vi "找搜索线上的分界点.vi"(6 "圆心":cluster{"X":sgl, "Y":sgl}, 9 "ROI 找边":T1 {"Contours"."Type" items=["No Selection", "Point", "Line", "Rectangle", "Oval", "Polygon", "Freehand Region", "Annulus", "Unused2", "Unused3", "Broken Line", "Freehand Line", "Rotated Rectangle"]}, 10 "Options":T3={"Edge Polarity"=2, "Kernel Size"=7, "Width"=7, "Minimum Edge Strength"=20.0, "Interpolation Type"=enum."Bilinear Fixed", "Data Processing Method"=enum."Average"} {"Edge Polarity" items=["All Edges", "Rising Edges", "Falling Edges"]; "Minimum Edge Strength" format="%.2f"; "Width" step=2; "Kernel Size" step=2}, 11 "引用句柄输入":T2) -> (0 "两点之间距离":sgl, 2 "Location (Pixel)":cluster{"X":sgl, "Y":sgl}, 3 "引用句柄输出":T2)   [LabVIEW 2014]
uses:
  <vilib>/vision/Measure.llb/Edge Options.ctl
  <vilib>/vision/Measure.llb/Edge Polarity.ctl
  <vilib>/vision/Image Controls.llb/IMAQ Image.ctl
  <vilib>/vision/NI_Vision_Development_Module.lvlib
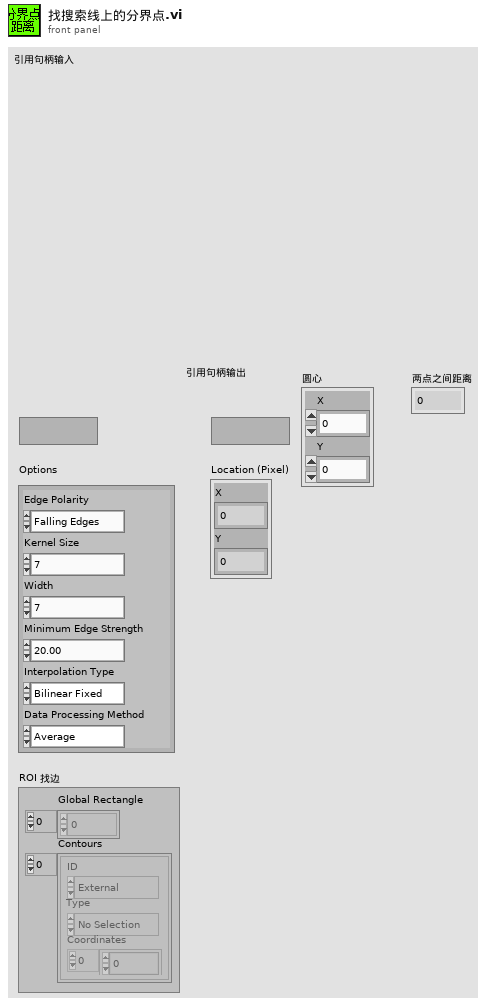
[diagram p1: front panel]
types:
  T1 = typedef "ROI Descriptor" = cluster{"Global Rectangle":i32[], "Contours":cluster{"ID":enum32{"External", "Internal"}, "Type":u32, "Coordinates":i32[]}[]}
  T2 = typedef "IMAQ Image.ctl" = refnum<image>
  T3 = typedef "Edge Options.ctl" = cluster{"Edge Polarity":T4, "Kernel Size":u32, "Width":u32, "Minimum Edge Strength":sgl, "Interpolation Type":enum32{"Zero Order", "Bilinear", "Quadratic", "Cubic", "Bilinear Fixed"}, "Data Processing Method":enum32{"Average", "Median"}}
  T4 = typedef "Edge Polarity.ctl" = u32
  T5 = enum16{"Get First Edge", "Get First + Last Edge", "Get All Edges", "Get Best Edge"}
  T6 = typedef "Edge New.ctl" = cluster{"Location (Pixel)":cluster{"X":sgl, "Y":sgl}, "Location (Real-World)":cluster{"X":sgl, "Y":sgl}, "Distance (Pixel)":dbl, "Distance (Real-World)":dbl, "Strength":dbl, "Noise":dbl, "Rising?":bool}
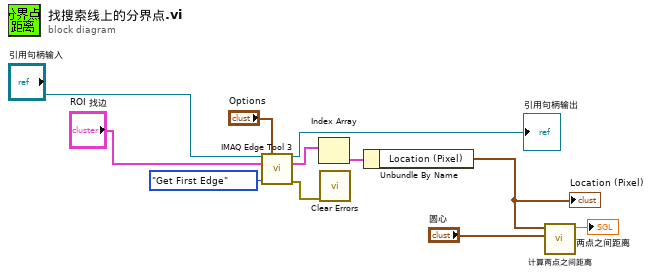
[diagram p0: block diagram]
diagram:
  n1 = call "IMAQ Edge Tool 3"("Image"="引用句柄输入", "Edge Options"="Options", "ROI Descriptor"="ROI 找边", "Process"=T5."Get First Edge") -> ("Image (duplicate)"=→"引用句柄输出":T2, "Edge Information"=w8:T6[], "error out"=w5:errorcluster)  [unwired: 7 in, 2 out]
  n2 = Index Array(array=w8) -> (element=w4:T6)  [unwired: 1 in]
  n3 = call <vilib>:"Clear Errors.vi"("error in (no error)"=w5) -> ()  [unwired: 5 in, 2 out]
  n4 = Unbundle By Name(w4) -> ("Location (Pixel)"=w3:cluster{"X":sgl, "Y":sgl})
  "Location (Pixel)" <- w3
  n5 = call "计算两点之间距离.vi"("Location (Pixel)"="圆心", "Center (Pixels)"=w3) -> ("两点之间距离"=→"两点之间距离":sgl)  [unwired: 9 in]
